vi "McPherson Set Slewing.vi"(0 "VISA Resource Name":refnum<visa-resource-name>, 2 "StepperPosition":i32 min=-8388607 max=8388607, 5 "error In":errorcluster, 7 "Old Slew":bool, 8 "Slew":bool, 10 "Previous ScanStatus":T1, 13 "Pause":bool) -> (12 "dup VISA Resource Name":refnum<visa-resource-name>, 14 "Continue?":bool, 16 "SlewStatus Out":T1, 18 "Speed out":i32 min=-100000 max=100000, 19 "error out":errorcluster)   [LabVIEW 2024]
uses:
  Globals and TypeDefs/Type Definitions.llb/McPherson Status.ctt
  Globals and TypeDefs/gSpectrometer.vi
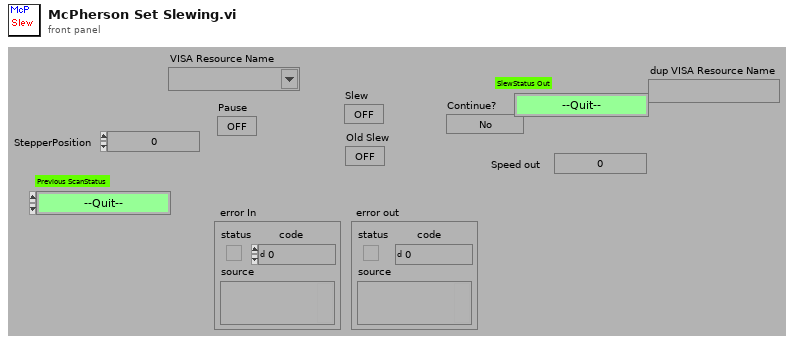
[diagram p1: front panel]
types:
  T1 = typedef "McPherson Status.ctt" = enum8{"--Quit--", "Error", "Initialization", "Standby", "Start Slew", "-Slew", "+Slew", "Slew Done", "Start Scan", "-Slew to Start", "+Slew to Start", "Scanning", "Scan Done", "Scan Pause", "Slew Pause", "Cancel", "Update Z0", "Sleep"}
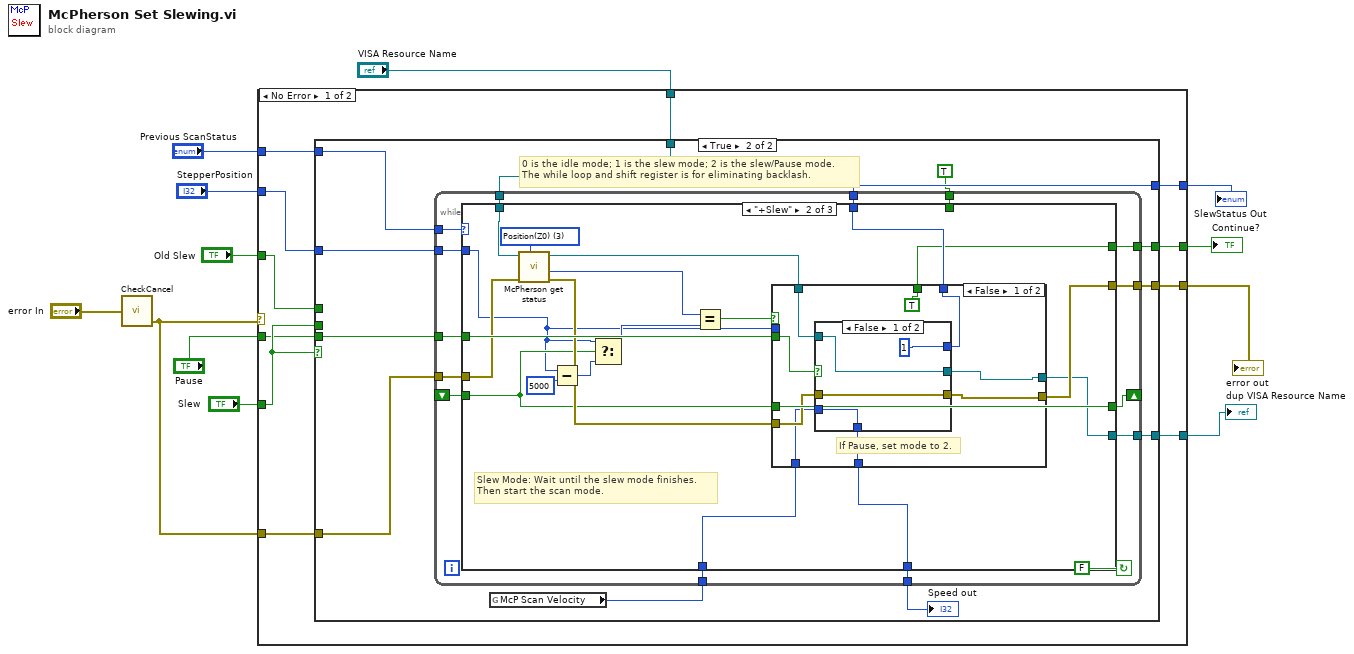
[diagram p0: block diagram]
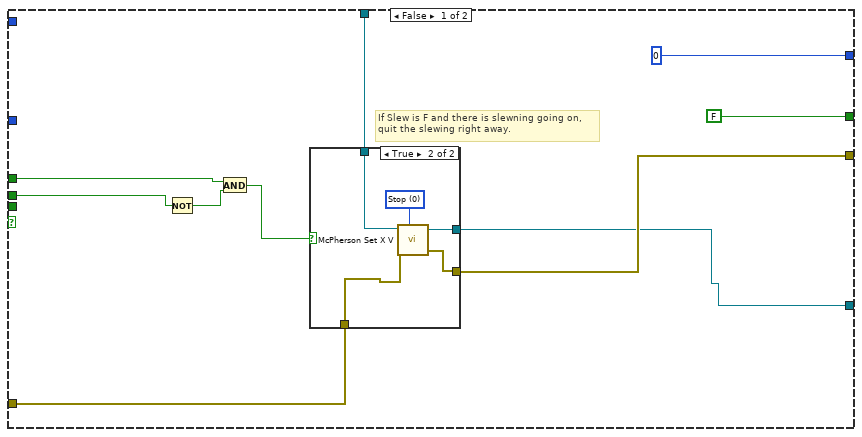
[diagram p2: hidden frame]
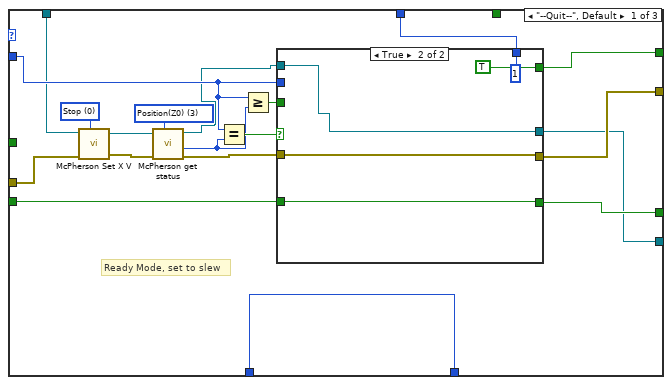
[diagram p4: hidden frame]
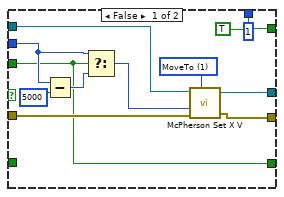
[diagram p5: hidden frame]
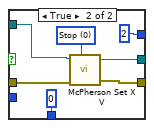
[diagram p6: hidden frame]
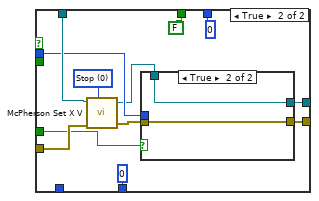
[diagram p7: hidden frame]
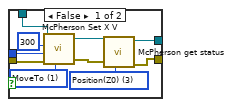
[diagram p8: hidden frame]
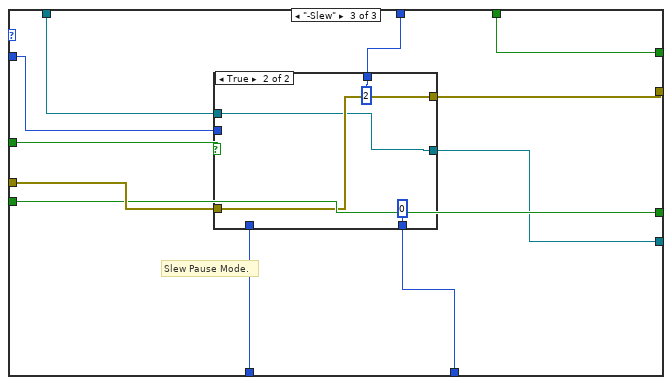
[diagram p9: hidden frame]
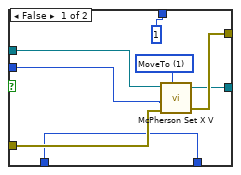
[diagram p10: hidden frame]
diagram:
  n1 = call "CheckCancel.vi"("error in (no error)"="error In") -> ("error out"=w1:errorcluster)  [unwired: 1 in, 1 out]
  n2 = case shown="No Error" w1 {
    tunnel: "VISA Resource Name" -> [w23 w190]
    tunnel: "Slew" -> [w22 _]
    tunnel: "Old Slew" -> [w21 w191]
    tunnel: [w20 w191] -> w10
    tunnel: "Pause" -> [w17 _]
    tunnel: "Previous ScanStatus" -> [w19 w193]
    tunnel: [w18 w193] -> w8
    tunnel: "StepperPosition" -> [w16 _]
    tunnel: w1 -> [w15 w192]
    tunnel: [w14 w192] -> w5
    tunnel: [w13 w190] -> w3
    frame No Error {
      n3 = case shown="True" w22 {
        tunnel: w16 -> [_ w44]
        tunnel: w23 -> [w32 w52]
        tunnel: w15 -> [w31 w51]
        tunnel: [w30 w50] -> w14
        tunnel: [FALSE w49] -> w20
        tunnel: w22 -> [w29 _]
        tunnel: w21 -> [w27 _]
        tunnel: w19 -> [_ w47]
        tunnel: [u8 0 ("ScanStatus") w46] -> w18
        tunnel: w17 -> [_ w45]
        tunnel: [w24 w42] -> w13
        frame False {
          # "If Slew is F and there is slewning going on,\nquit the slewing right away."
          n4 = Not(x=w29) -> (.not. x?=w28:bool)
          n5 = And(x=w27, y=w28) -> (x .and. y?=w26:bool)
          n6 = case shown="True" w26 {
            tunnel: w32 -> [w34 w40]
            tunnel: w31 -> [w35 w39]
            tunnel: [w35 w38] -> w30
            tunnel: [w34 w36] -> w24
            frame False {
            }
            frame True {
              w37 = u8 0 items=["Stop", "MoveTo", "SpeedAt"] ("Action")
              n7 = call "McPherson Set X V.vi"("VISA Resource Name"=w40, "error In"=w39, "Action"=w37) -> ("dup VISA Resource Name"=w36:refnum<visa-resource-name>, "error out"=w38:errorcluster)  [unwired: 2 in, 1 out]
            }
          }
        }
        frame True {
          # "0 is the idle mode; 1 is the slew mode; 2 is the slew/Pause mode.\nThe while loop and shift register is for eliminating backlash."
          n8 = global read "gSpectrometer.vi" "McP Scan Velocity"() -> (w41:i32)
          n9 = while {
            shift-left: _ -> [w55]
            shift-right: [w56] -> _
            tunnel: TRUE ("Ramp") -> [w57]
            tunnel: w41 -> [w58]
            tunnel: w44 -> [w59]
            tunnel: w45 -> [w60]
            tunnel: [w61] -> w46
            tunnel: w47 -> [w62]
            tunnel: [w63] -> w48
            tunnel: [w64] -> w49
            tunnel: [w65] -> w50
            tunnel: w51 -> [w66]
            tunnel: w52 -> [w67]
            tunnel: [w53] -> w42
            stop <- FALSE continue-if-true
            n10 = case shown="\"+Slew\"" w62 {
              tunnel: w67 -> [w71 w106 w176]
              tunnel: w59 -> [w74 w107 w177]
              tunnel: w66 -> [w84 w115 w172]
              tunnel: [w85 w122 w175] -> w65
              tunnel: [w78 w117 w171] -> w64
              tunnel: [w86 w118 w169] -> w63
              tunnel: [w79 w119 w174] -> w61
              tunnel: w60 -> [_ w120 w173]
              tunnel: w58 -> [w86 w112 w170]
              tunnel: w57 -> [_ _ w171]
              tunnel: [w73 w108 w168] -> w56
              tunnel: w55 -> [w72 w108 w168]
              tunnel: [w68 w104 w167] -> w53
              frame "--Quit--", Default {
                w82 = u16 3 items=["Grab Globals", "Full (X, ^, Z0)", "Moving(^ and Z0)", "Position(Z0)"] ("Status")
                w83 = u8 0 items=["Stop", "MoveTo", "SpeedAt"] ("Action")
                # "Ready Mode, set to slew"
                n11 = call "McPherson Set X V.vi"("VISA Resource Name"=w71, "error In"=w84, "Action"=w83) -> ("dup VISA Resource Name"=w70:refnum<visa-resource-name>, "error out"=w81:errorcluster)  [unwired: 2 in, 1 out]
                n12 = call "McPherson get status.vi"("Status"=w82, "error in (no error)"=w81, "VISA Resource Name"=w70) -> ("error out"=w80:errorcluster, "CurrentPosition"=w76:i32, "dup VISA Resource Name"=w69:refnum<visa-resource-name>)  [unwired: 2 in, 1 out]
                n13 = Equal?(x=w74, y=w76) -> (x = y?=w77:bool)
                n14 = Greater Or Equal?(x=w74, y=w76) -> (x >= y?=w75:bool)
                n15 = case shown="True" w77 {
                  tunnel: [w98 w101] -> w85
                  tunnel: w69 -> [w96 w99]
                  tunnel: w80 -> [w95 w101]
                  tunnel: [u8 1 ("ScanStatus") u8 1 ("ScanStatus")] -> w79
                  tunnel: [TRUE ("Ramp") TRUE ("Ramp")] -> w78
                  tunnel: w75 -> [w88 _]
                  tunnel: w74 -> [w91 _]
                  tunnel: [w88 w100] -> w73
                  tunnel: w72 -> [_ w100]
                  tunnel: [w87 w99] -> w68
                  frame False {
                    w97 = u8 1 items=["Stop", "MoveTo", "SpeedAt"] ("Action")
                    n16 = Subtract(x=w91, y=5000) -> (x-y=w90:i32)
                    n17 = Select(t=w91, s=w88, f=w90) -> (s? t:f=w92:i32)
                    n18 = call "McPherson Set X V.vi"("VISA Resource Name"=w96, "SetValue In"=w92, "error In"=w95, "Action"=w97) -> ("dup VISA Resource Name"=w87:refnum<visa-resource-name>, "error out"=w98:errorcluster)  [unwired: 1 in, 1 out]
                  }
                  frame True {
                  }
                }
              }
              frame "+Slew" {
                w114 = u16 3 items=["Grab Globals", "Full (X, ^, Z0)", "Moving(^ and Z0)", "Position(Z0)"] ("Status")
                # "Slew Mode: Wait until the slew mode finishes.\nThen start the scan mode."
                n19 = call "McPherson get status.vi"("Status"=w114, "error in (no error)"=w115, "VISA Resource Name"=w106) -> ("error out"=w116:errorcluster, "CurrentPosition"=w113:i32, "dup VISA Resource Name"=w105:refnum<visa-resource-name>)  [unwired: 2 in, 1 out]
                n20 = Subtract(x=w107, y=5000) -> (x-y=w110:i32)
                n21 = Select(t=w107, s=w108, f=w110) -> (s? t:f=w109:i32)
                n22 = Equal?(x=w113, y=w109) -> (x = y?=w121:bool)
                n23 = case shown="False" w121 {
                  tunnel: w105 -> [w127 w147]
                  tunnel: w116 -> [w128 w150]
                  tunnel: [w129 w148] -> w122
                  tunnel: [w125 0 ("McP Scan Velocity")] -> w118
                  tunnel: [w130 u8 0 ("ScanStatus")] -> w119
                  tunnel: w120 -> [w131 _]
                  tunnel: w112 -> [w126 _]
                  tunnel: [TRUE ("Ramp") FALSE ("Ramp")] -> w117
                  tunnel: w108 -> [_ w146]
                  tunnel: w107 -> [_ w145]
                  tunnel: [w123 w143] -> w104
                  frame False {
                    # "If Pause, set mode to 2."
                    n24 = case shown="False" w131 {
                      tunnel: [u8 1 ("ScanStatus") u8 2 ("ScanStatus")] -> w130
                      tunnel: [w134 w142] -> w129
                      tunnel: w128 -> [w134 w141]
                      tunnel: w127 -> [w132 w139]
                      tunnel: w126 -> [w133 _]
                      tunnel: [w133 0 ("McP Scan Velocity")] -> w125
                      tunnel: [w132 w136] -> w123
                      frame False {
                      }
                      frame True {
                        w138 = u8 0 items=["Stop", "MoveTo", "SpeedAt"] ("Action")
                        n25 = call "McPherson Set X V.vi"("VISA Resource Name"=w139, "error In"=w141, "Action"=w138) -> ("dup VISA Resource Name"=w136:refnum<visa-resource-name>, "error out"=w142:errorcluster)  [unwired: 2 in, 1 out]
                      }
                    }
                  }
                  frame True {
                    w151 = u8 0 items=["Stop", "MoveTo", "SpeedAt"] ("Action")
                    n26 = call "McPherson Set X V.vi"("VISA Resource Name"=w147, "error In"=w150, "Action"=w151) -> ("dup VISA Resource Name"=w144:refnum<visa-resource-name>, "error out"=w149:errorcluster)  [unwired: 2 in, 1 out]
                    n27 = case shown="True" w146 {
                      tunnel: [w161 w166] -> w148
                      tunnel: w149 -> [w164 w166]
                      tunnel: w144 -> [w157 w165]
                      tunnel: w145 -> [w163 _]
                      tunnel: [w155 w165] -> w143
                      frame False {
                        w159 = u8 1 items=["Stop", "MoveTo", "SpeedAt"] ("Action")
                        w160 = u16 3 items=["Grab Globals", "Full (X, ^, Z0)", "Moving(^ and Z0)", "Position(Z0)"] ("Status")
                        n28 = call "McPherson Set X V.vi"("VISA Resource Name"=w157, "milliseconds to wait"=u32 300, "SetValue In"=w163, "error In"=w164, "Action"=w159) -> ("dup VISA Resource Name"=w156:refnum<visa-resource-name>, "error out"=w162:errorcluster)  [unwired: 1 out]
                        n29 = call "McPherson get status.vi"("Status"=w160, "error in (no error)"=w162, "VISA Resource Name"=w156) -> ("error out"=w161:errorcluster, "dup VISA Resource Name"=w155:refnum<visa-resource-name>)  [unwired: 2 in, 2 out]
                      }
                      frame True {
                      }
                    }
                  }
                }
              }
              frame "-Slew" {
                # "Slew Pause Mode."
                n30 = case shown="True" w173 {
                  tunnel: w177 -> [w181 _]
                  tunnel: w176 -> [w182 w186]
                  tunnel: [w185 w189] -> w175
                  tunnel: [u8 1 ("ScanStatus") u8 2 ("ScanStatus")] -> w174
                  tunnel: w172 -> [w183 w189]
                  tunnel: [w179 0 ("McP Scan Velocity")] -> w169
                  tunnel: w170 -> [w179 _]
                  tunnel: [w178 w186] -> w167
                  frame False {
                    w180 = u8 1 items=["Stop", "MoveTo", "SpeedAt"] ("Action")
                    n31 = call "McPherson Set X V.vi"("VISA Resource Name"=w182, "SetValue In"=w181, "error In"=w183, "Action"=w180) -> ("dup VISA Resource Name"=w178:refnum<visa-resource-name>, "error out"=w185:errorcluster)  [unwired: 1 in, 1 out]
                  }
                  frame True {
                  }
                }
              }
            }
          }
          "Speed out" <- w48
        }
      }
    }
    frame Error {
    }
  }
  "SlewStatus Out" <- w8
  "Continue?" <- w10
  "error out" <- w5
  "dup VISA Resource Name" <- w3
